vi "Type to String.vi"(10 "Data Type":T1) -> (2 "String Type":string)   [LabVIEW 2019, in "UDP-Custom-Device Shared.lvlib"]
uses:
  UDP-Custom-Device Shared.lvlib
  Types/Shared - Channel Data Type.ctl
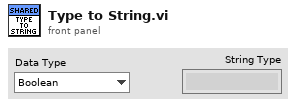
[diagram p1: front panel]
types:
  T1 = typedef "UDP-Custom-Device Shared.lvlib/Shared - Channel Data Type.ctl" = enum16{"Boolean", "Single", "Double", "I8", "I16", "I32", "I64", "U8", "U16", "U32", "U64"}
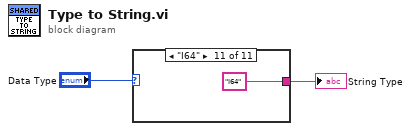
[diagram p0: block diagram]
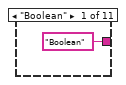
[diagram p2: hidden frame]
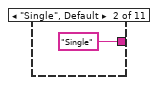
[diagram p3: hidden frame]
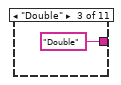
[diagram p4: hidden frame]
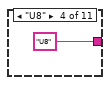
[diagram p5: hidden frame]
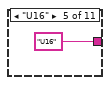
[diagram p6: hidden frame]
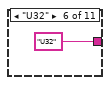
[diagram p7: hidden frame]
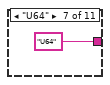
[diagram p8: hidden frame]
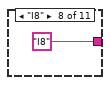
[diagram p9: hidden frame]
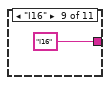
[diagram p10: hidden frame]
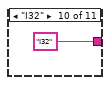
[diagram p11: hidden frame]
diagram:
  n1 = case shown="\"I64\"" "Data Type" {
    tunnel: ["Boolean" "Single" "Double" "U8" "U16" "U32" "U64" "I8" "I16" "I32" "I64"] -> w1
    frame "Boolean" {
    }
    frame "Single", Default {
    }
    frame "Double" {
    }
    frame "U8" {
    }
    frame "U16" {
    }
    frame "U32" {
    }
    frame "U64" {
    }
    frame "I8" {
    }
    frame "I16" {
    }
    frame "I32" {
    }
    frame "I64" {
    }
  }
  "String Type" <- w1
